vi "TestCallingPy.vi"() -> ()   [LabVIEW 2024]
panel:
  out "Array":T1(array[cluster])
  out "value":T2
  out "return value":string
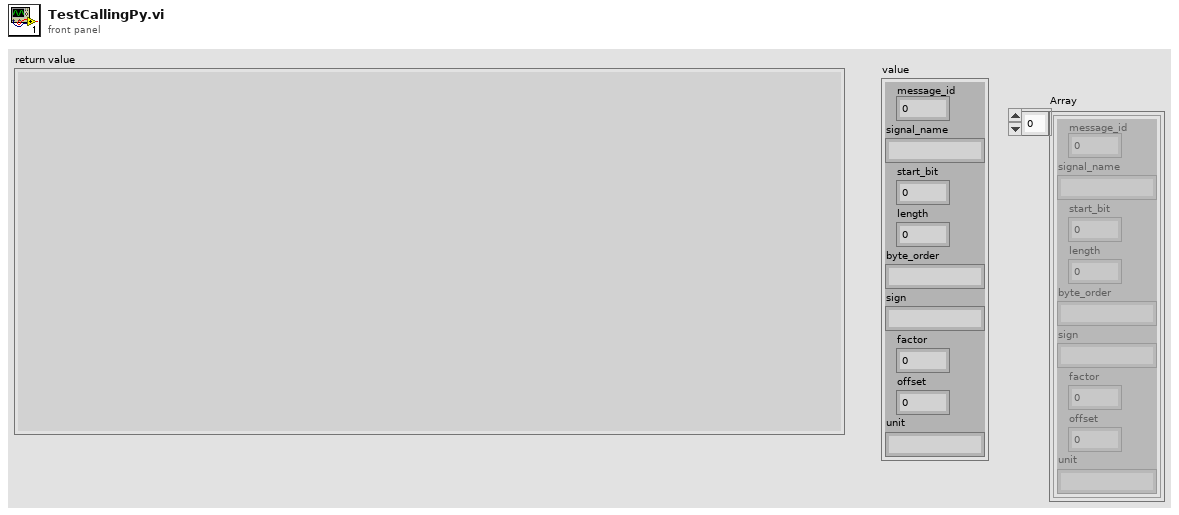
[diagram p1: front panel]
types:
  T1 = cluster{"message_id":i32, "signal_name":string, "start_bit":i32, "length":i32, "byte_order":string, "sign":string, "factor":dbl, "offset":dbl, "unit":string}[]
  T2 = cluster{"message_id":i32, "signal_name":string, "start_bit":i32, "length":i32, "byte_order":string, "sign":string, "factor":dbl, "offset":dbl, "unit":string}
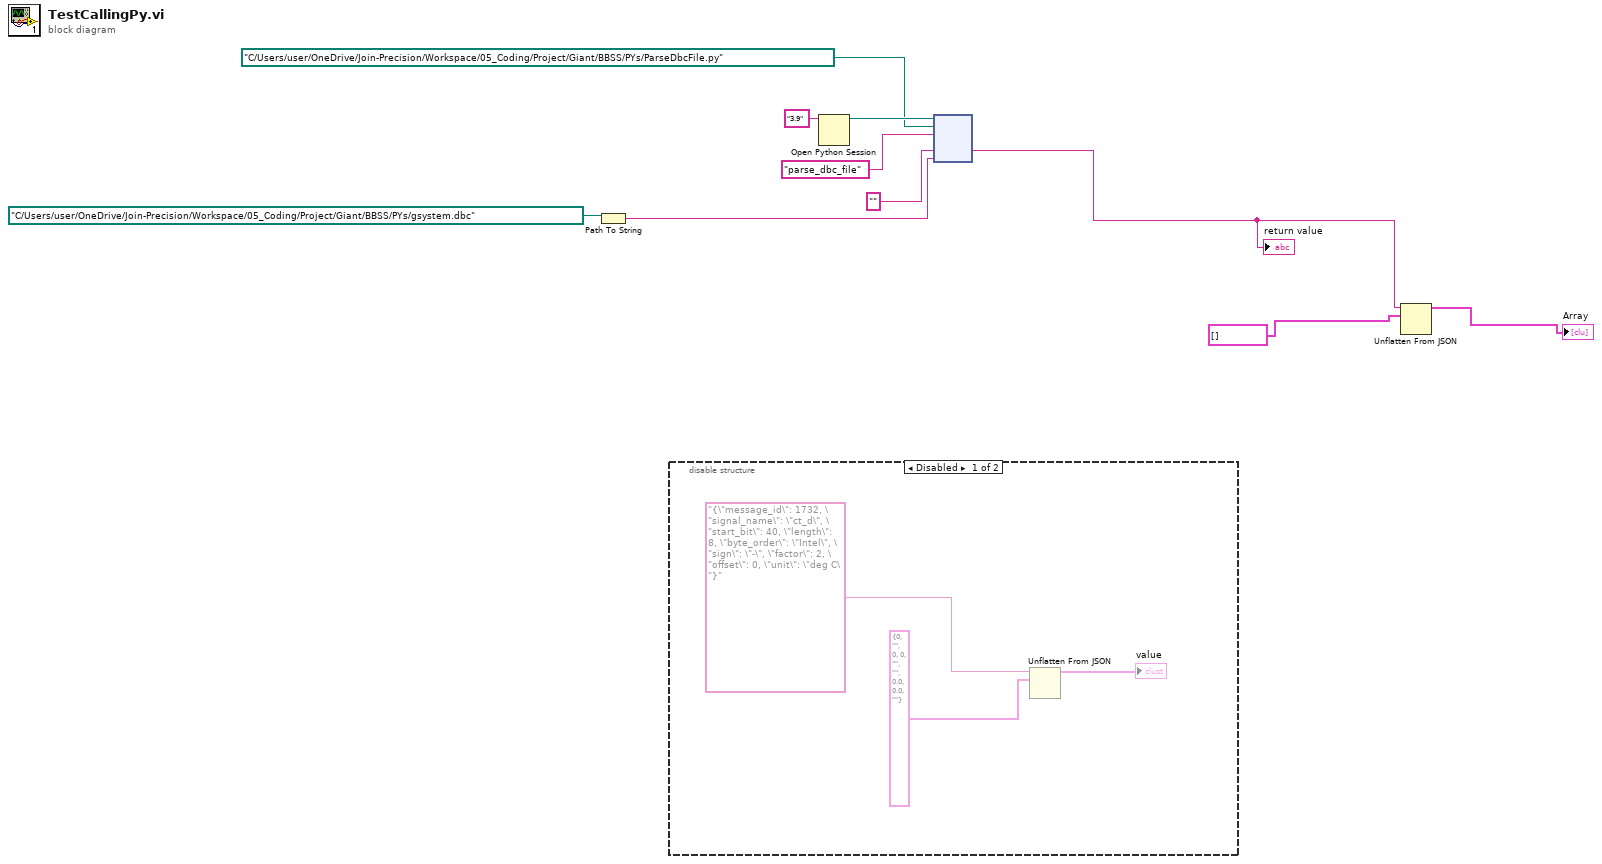
[diagram p0: block diagram]
diagram:
  n1 = Path To String(path=path "C:/Users/user/OneDrive/Join-Precision/Workspace/05_Coding/Project/Giant/BBSS/PYs/gsystem.dbc") -> (string=w5:string)
  n2 = disable-structure shown="Disabled" {
    frame Disabled {
      n3 = Unflatten From JSON(JSON string="{\"message_id\": 1732, \"signal_name\": \"ct_d\", \"start_bit\": 40, \"length\": 8, \"byte_order\": \"Intel\", \"sign\": \"-\", \"factor\": 2, \"offset\": 0, \"unit\": \"deg C\"}", type and defaults=T2 {"message_id"=0, "signal_name"="", "start_bit"=0, "length"=0, "byte_order"="", "sign"="", "factor"=0.0, "offset"=0.0, "unit"=""} ("value")) -> (value=→"value":T2)  [unwired: 5 in, 1 out]
    }
    frame Enabled {
    }
  }
  n4 = Open Python Session(python version="3.9" ("Python version")) -> (session out=w9:refnum<k35>)  [unwired: 2 in, 1 out]
  n5 = node(w9, path "C:/Users/user/OneDrive/Join-Precision/Workspace/05_Coding/Project/Giant/BBSS/PYs/ParseDbcFile.py" ("module path"), "parse_dbc_file" ("function name"), "", w5) -> (w1:string)  [unwired: 2 in, 4 out]
  "return value" <- w1
  n6 = Unflatten From JSON(JSON string=w1, type and defaults=T1 [] ("Array")) -> (value=→"Array":T1)  [unwired: 5 in, 1 out]
